vi "Read id.vi"(8 "error in (no error)":errorcluster, 11 "DSFPluginSettings in":refnum<class "DSFPluginSettings.lvclass">) -> (0 "error out":errorcluster, 2 "id":string, 3 "DSFPluginSettings out":refnum<class "DSFPluginSettings.lvclass">)   [LabVIEW 2017, in "DSFPluginSettings.lvclass"]
uses:
  DSFPluginSettings.lvclass
  DSFPluginSettings.lvclass/DSFPluginSettings.ctl
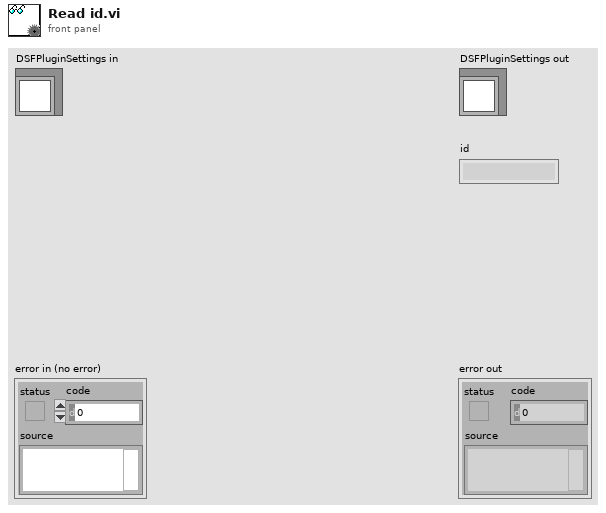
[diagram p1: front panel]
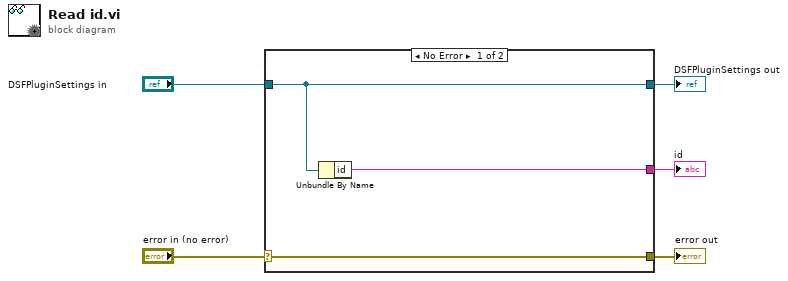
[diagram p0: block diagram]
diagram:
  n1 = case shown="No Error" "error in (no error)" {
    selector: "error in (no error)" -> [w8 w9]
    tunnel: [w8 w9] -> w4
    tunnel: [w7 w10] -> w2
    tunnel: "DSFPluginSettings in" -> [w7 w10]
    tunnel: [w6 _] -> w1
    frame No Error {
      n2 = Unbundle By Name(w7) -> ("id"=w6:string)
    }
    frame Error {
    }
  }
  "error out" <- w4
  "DSFPluginSettings out" <- w2
  "id" <- w1
